vi "VI-Create Reference Array Dialog.vi"   [LabVIEW 2015]
panel:
  # "Creating reference array..."
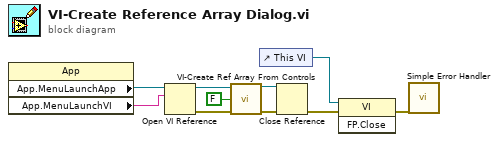
[diagram p0: block diagram]
diagram:
  n1 = property class="App"() -> ("App.MenuLaunchApp"=w10:refnum<vi>, "App.MenuLaunchVI"=w9:string)  [unwired: 2 in, 2 out]
  n2 = Open VI Reference(application reference (local)=w10, vi path=w9) -> (vi reference=w8:refnum<vi>, error out=w6:errorcluster)  [unwired: 4 in]
  n3 = call "VI-Create Ref Array From Controls.vi"("VI ref in"=w8, "Create typedef?"=FALSE, "error in (no error)"=w6) -> ("VI ref out"=w4:refnum<vi>, "error out"=w5:errorcluster)  [unwired: 8 in, 3 out]
  n4 = control-ref of="This VI"() -> (w3:refnum<vi>)
  n5 = Close Reference(reference=w4, error in (no error)=w5) -> (error out=w2:errorcluster)
  n6 = invoke class="VI" method="FP.Close"(reference=w3, error in=w2) -> (error out=w1:errorcluster)  [unwired: 1 in, 2 out]
  n7 = call <vilib>:"Simple Error Handler.vi"("error in (no error)"=w1) -> ()  [unwired: 4 in, 5 out]
